vi "PutIDCard.vi"() -> (2 "ID_CARD":string)   [LabVIEW 2018]
panel:
  in  "Finalizar":bool
  in  "Usuario(numero de tarjeta):":string
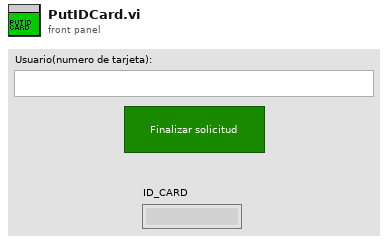
[diagram p1: front panel]
types:
  T1 = enum32{"Invalid", "Standard", "Closed", "Hidden", "Minimized", "Maximized"}
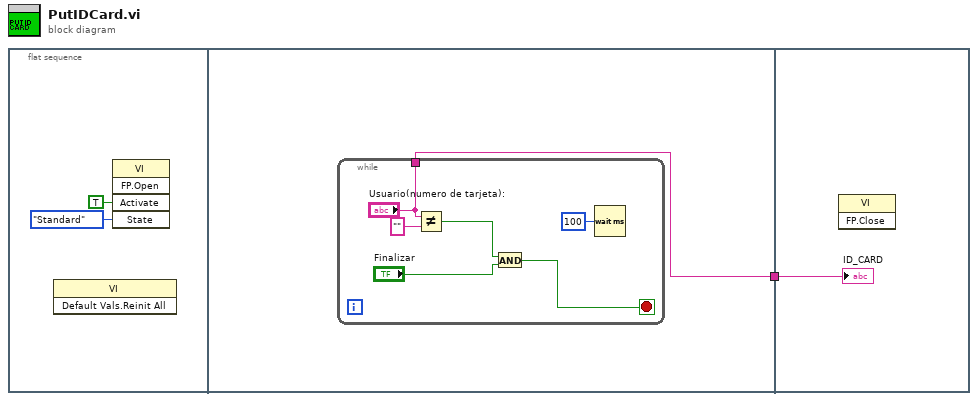
[diagram p0: block diagram]
diagram:
  n1 = flat-sequence {
    tunnel: [w4] -> w1
    tunnel: w1 -> [w11]
    frame #0 {
      n2 = invoke class="VI" method="Default Vals.Reinit All"() -> ()  [unwired: 3 in, 3 out]
      n3 = invoke class="VI" method="FP.Open"("Activate"=TRUE ("Activate?"), "State"=T1."Standard") -> ()  [unwired: 3 in, 5 out]
    }
    frame #1 {
      n4 = while {
        tunnel: ["Usuario(numero de tarjeta):"] -> w4
        stop <- w7 stop-if-true
        n5 = Not Equal?(x="Usuario(numero de tarjeta):", y="") -> (x != y?=w8:bool)
        n6 = And(x=w8, y="Finalizar") -> (x .and. y?=w7:bool)
        n7 = Wait (ms)(milliseconds to wait=u32 100) -> ()  [unwired: 1 out]
      }
    }
    frame #2 {
      n8 = invoke class="VI" method="FP.Close"() -> ()  [unwired: 3 in, 3 out]
      "ID_CARD" <- w11
    }
  }
